vi "Test_WriteValue_InvalidType_Error.vi"(8 "error in (no error)":errorcluster, 11 "TestCase in":refnum<class "TestTerminalCaptionBinding.lvclass">) -> (0 "error out":errorcluster, 3 "TestCase out":refnum<class "TestTerminalCaptionBinding.lvclass">)   [LabVIEW 2017, in "TestTerminalCaptionBinding.lvclass"]
uses:
  TestTerminalCaptionBinding.lvclass
  Source/Concrete/TerminalCaptionBinding/TerminalCaptionBinding.lvclass
  C:/Git/composed-transport/Source/ITransport/ITransport.lvclass
  Source/ITransport/ITransport.lvclass
panel:
  out "Return Error":errorcluster
  in  "Numeric":dbl
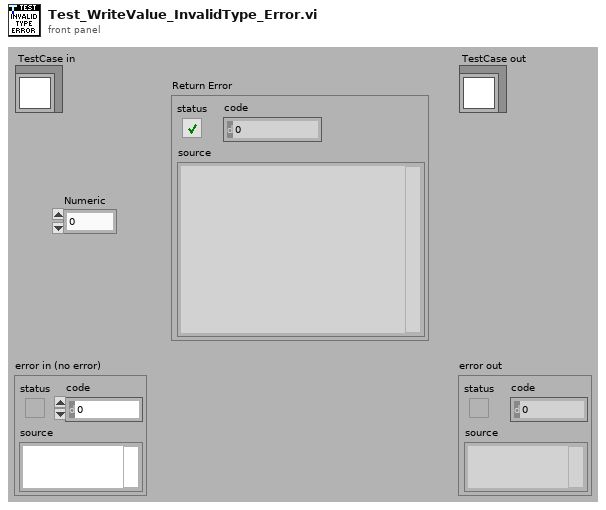
[diagram p1: front panel]
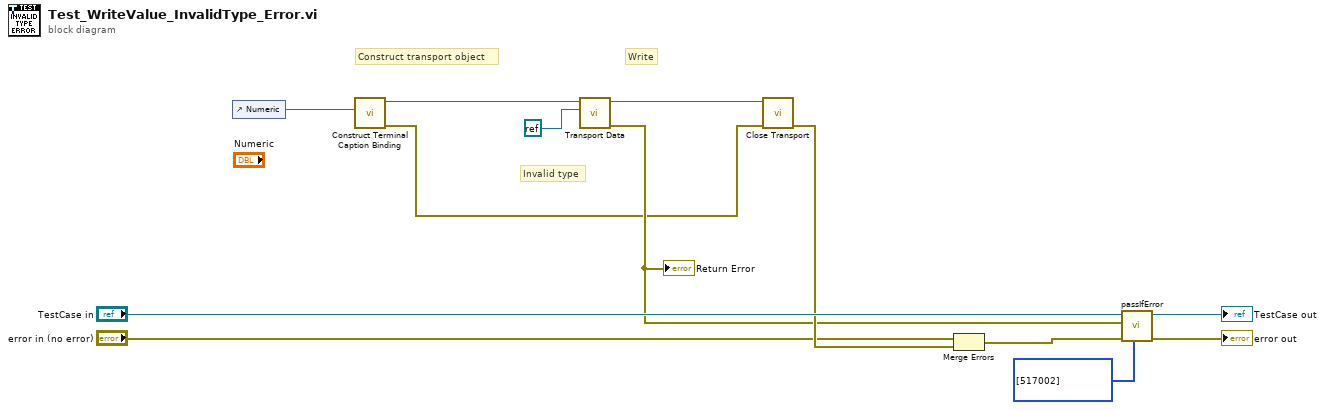
[diagram p0: block diagram]
diagram:
  # "Invalid type"
  # "Write"
  # "Construct transport object"
  n1 = control-ref of="Numeric"() -> (w9:refnum<vi>)
  n2 = call "Construct Terminal Caption Binding.vi"("Ctl Refnum"=w9) -> ("error out"=w3:errorcluster, "TerminalCaptionBinding"=w10:refnum<class "TerminalCaptionBinding.lvclass">)  [unwired: 9 in]
  n3 = call "Transport Data.vi"("Value"=refnum<k0> refnum, "ITransport in"=w10) -> ("error out"=w6:errorcluster, "ITransport out"=w7:refnum<class "TerminalCaptionBinding.lvclass">)  [unwired: 8 in]
  "Return Error" <- w6
  n4 = call-dynamic "Close Transport.vi"("error in (no error)"=w3, "ITransport in"=w7) -> ("error out"=w8:errorcluster)  [unwired: 9 in]
  n5 = Merge Errors("error in (no error)", w8) -> (w2:errorcluster)
  n6 = call-dynamic "passIfError.vi"("passing error codes (default = any error code)"=i32[] [517002], "error in (no error)"=w2, "error"=w6, "TestCase in"="TestCase in") -> ("error out"=→"error out":errorcluster, "TestCase out"=→"TestCase out":refnum<class "TestTerminalCaptionBinding.lvclass">)  [unwired: 6 in]
